vi "IT6700H Output DC Volts.vi"() -> ()   [LabVIEW 2015]
uses:
  <instrlib>/IT6700H/IT6700H.lvlib
panel:
  in  "Serial Configuration":T1={"Baud Rate"=9600, "Parity"=0, "Data Bits"=8, "Stop Bits"=10, "Flow Control"=0} {"Flow Control" items=["None", "XON/XOFF", "RTS/CTS", "XON/XOFF & RTS/CTS", "DTR/DSR", "XON/XOFF & DTR/DSR"]; "Stop Bits" items=["1.0"=10, "1.5"=15, "2.0"=20]; "Data Bits" items=["7"=7, "8"=8]; "Parity" items=["None", "Odd", "Even", "Mark", "Space"]; "Baud Rate" items=["300"=300, "600"=600, "1200"=1200, "2400"=2400, "4800"=4800, "9600"=9600, "19200"=19200]}
  in  "Stop Output":bool
  in  "Voltage Level (0V)":dbl=3.0 format="%.2f"
  out "Actual Current Level (A)":dbl format="%.3f"
  out "Actual Voltage Level (V)":dbl format="%.3f"
  in  "Current Level (0A)":dbl=1.0 format="%.2f"
  in  "VISA resource name":refnum<visa-resource-name>
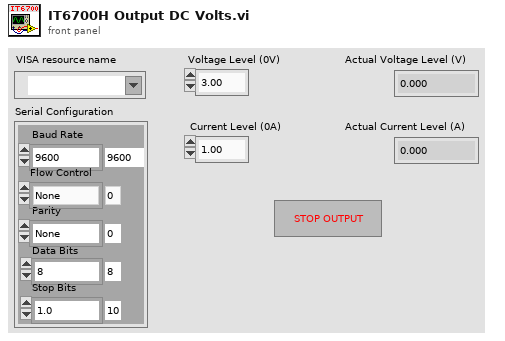
[diagram p1: front panel]
types:
  T1 = cluster{"Baud Rate":u32, "Parity":u16, "Data Bits":u16, "Stop Bits":u16, "Flow Control":u16}
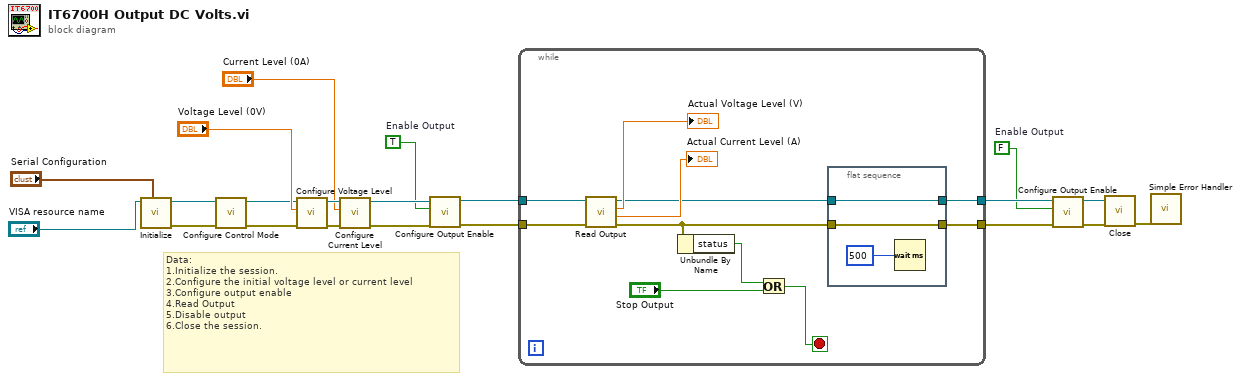
[diagram p0: block diagram]
diagram:
  w8 = FALSE  # Enable Output
  w9 = TRUE  # Enable Output
  # "Data:\n1.Initialize the session.\n2.Configure the initial voltage level or current level\n3.Configure output enable\n4.Read Output\n5.Disable output\n6.Close the session."
  n1 = call <instrlib>:"Initialize.vi"("Serial Configuration"="Serial Configuration", "VISA resource name"="VISA resource name") -> ("error out"=w2:errorcluster, "VISA resource name out"=w4:refnum<visa-resource-name>)  [unwired: 8 in]
  n2 = call <instrlib>:"Configure Control Mode.vi"("error in (no error)"=w2, "VISA resource name"=w4) -> ("error out"=w1:errorcluster, "VISA resource name out"=w3:refnum<visa-resource-name>)  [unwired: 8 in]
  n3 = call <instrlib>:"Configure Voltage Level.vi"("error in (no error)"=w1, "Voltage Level (0.0 V)"="Voltage Level (0V)", "VISA resource name"=w3) -> ("error out"=w18:errorcluster, "VISA resource name out"=w17:refnum<visa-resource-name>)  [unwired: 7 in]
  n4 = call <instrlib>:"Configure Current Level.vi"("error in (no error)"=w18, "Current Level (0.0 A)"="Current Level (0A)", "VISA resource name"=w17) -> ("error out"=w14:errorcluster, "VISA resource name out"=w15:refnum<visa-resource-name>)  [unwired: 7 in]
  n5 = call <instrlib>:"Configure Output Enable.vi"("VISA resource name"=w15, "Enable Output (T: Enable)"=w9, "error in (no error)"=w14) -> ("VISA resource name out"=w13:refnum<visa-resource-name>, "error out"=w12:errorcluster)  [unwired: 6 in]
  n6 = while {
    tunnel: w13 -> [w32]
    tunnel: w12 -> [w31]
    tunnel: [w25] -> w11
    tunnel: [w22] -> w10
    stop <- w26 stop-if-true
    n7 = call <instrlib>:"Read Output.vi"("error in (no error)"=w31, "VISA resource name"=w32) -> ("error out"=w23:errorcluster, "Actual Current Level (A)"=→"Actual Current Level (A)":dbl, "Actual Voltage Level (V)"=→"Actual Voltage Level (V)":dbl, "VISA resource name out"=w24:refnum<visa-resource-name>)  [unwired: 6 in]
    n8 = Unbundle By Name(w23) -> ("status"=w28:bool)
    n9 = Or(x=w28, y="Stop Output") -> (x .or. y?=w26:bool)
    n10 = flat-sequence {
      tunnel: [w35] -> w25
      tunnel: w24 -> [w35]
      tunnel: [w34] -> w22
      tunnel: w23 -> [w34]
      frame #0 {
        n11 = Wait (ms)(milliseconds to wait=500) -> ()  [unwired: 1 out]
      }
    }
  }
  n12 = call <instrlib>:"Configure Output Enable.vi"("VISA resource name"=w11, "Enable Output (T: Enable)"=w8, "error in (no error)"=w10) -> ("VISA resource name out"=w6:refnum<visa-resource-name>, "error out"=w7:errorcluster)  [unwired: 6 in]
  n13 = call <instrlib>:"Close.vi"("error in (no error)"=w7, "VISA resource name"=w6) -> ("error out"=w5:errorcluster)  [unwired: 9 in]
  n14 = call <vilib>:"Simple Error Handler.vi"("error in (no error)"=w5) -> ()  [unwired: 4 in, 5 out]
